vi "Create AP Sx Menu.vi"(6 "beforeMenuItemID":i32, 7 "beforeMenuID":i32, 8 "error in (no error)":errorcluster caption="错误输入（无错误）", 9 "menuBarHandle":i32, 10 "panelHandle":i32, 11 "asicHandle":i32) -> (0 "error out":errorcluster caption="错误输出", 3 "function return":i32)   [LabVIEW 2018]
doc: "extern int __stdcall CreateAPSxMenu (int asicHandle, IN int panelHandle, IN int menuBarHandle, IN int beforeMenuID, IN int beforeMenuItemID);"
uses:
  APSx.dll/APSx.dll
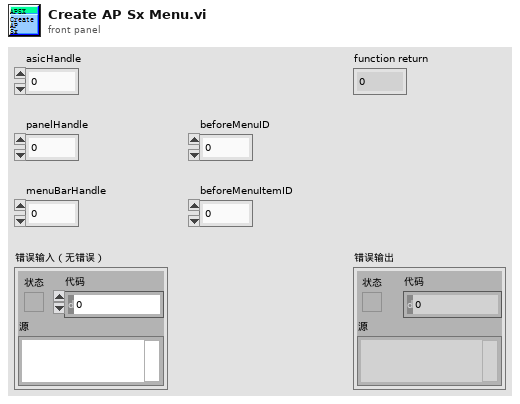
[diagram p1: front panel]
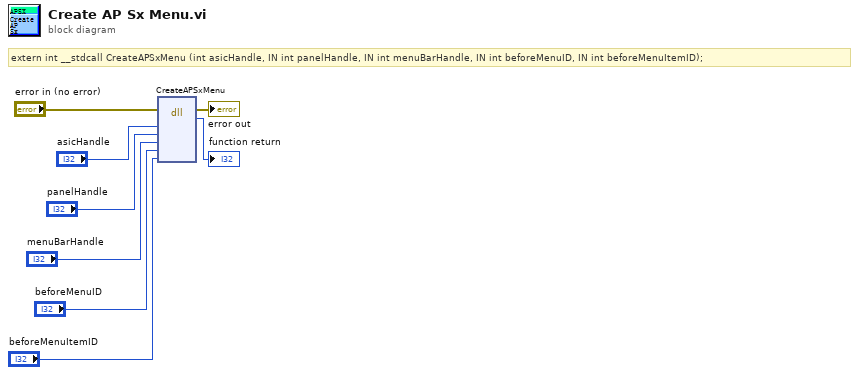
[diagram p0: block diagram]
diagram:
  # "extern int __stdcall CreateAPSxMenu (int asicHandle, IN int panelHandle, IN int menuBarHandle, IN int beforeMenuID, IN int beforeMenuItemID);"
  n1 = dll-call lib="PTH2[abs D项目Feng恒隆项目Labview传感器对中台SourcesAPSx.dllAPSx.*" fn="CreateAPSxMenu"(error in="error in (no error)", "asicHandle"="asicHandle", "panelHandle"="panelHandle", "menuBarHandle"="menuBarHandle", "beforeMenuID"="beforeMenuID", "beforeMenuItemID"="beforeMenuItemID") -> (error out=→"error out":errorcluster, →"function return":i32)  [unwired: 7 in, 1 out]
